vi "fileAsynchronousCreate.vi"   [LabVIEW 2017]
uses:
  globalUtilities.vi
types:
  T1 = enum16{"open", "replace", "create", "open or create", "replace or create", "replace or create with confirmation"}
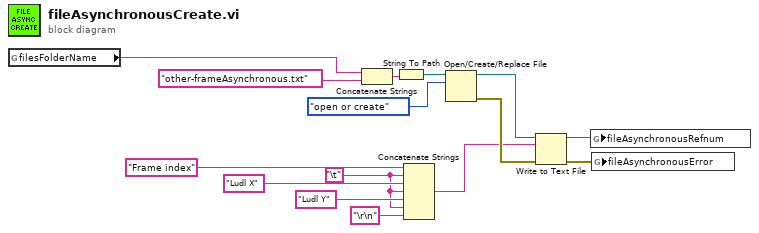
[diagram p0: block diagram]
diagram:
  w2 = "\t"
  n1 = global read "globalUtilities.vi" "filesFolderName"() -> (w6:string)
  n2 = Concatenate Strings(w6, "other-frameAsynchronous.txt") -> (w14:string)
  n3 = String To Path(string=w14) -> (path=w13:path)
  n4 = Concatenate Strings("Frame index" ("string"), w2, "Ludl X" ("string"), w2, "Ludl Y" ("string"), w2, "\r\n" ("string")) -> (w7:string)
  n5 = Open/Create/Replace File(file path (use dialog)=w13, operation (0:open)=T1."open or create") -> (refnum out=w11:refnum<file>, error out=w10:errorcluster)  [unwired: 4 in, 1 out]
  n6 = Write to Text File(file (use dialog)=w11, text=w7, error in=w10) -> (refnum out=w5:refnum<file>, error out=w4:errorcluster)  [unwired: 1 in, 1 out]
  n7 = global write "globalUtilities.vi" "fileAsynchronousRefnum"(w5) -> ()
  n8 = global write "globalUtilities.vi" "fileAsynchronousError"(w4) -> ()
